vi "Pasive Response to IP & Port.vi"(8 "error in (no error)":errorcluster, 10 "Response":string, 11 "FTP in":refnum<class "FTP.lvclass">) -> (0 "error out":errorcluster, 1 "Port":u16, 2 "IP":u32 format="%x", 3 "FTP out":refnum<class "FTP.lvclass">)   [LabVIEW 2020, in "FTP.lvlib" / "FTP.lvclass"]
uses:
  FTP.lvclass
panel:
  out "array":u32[](array[numeric]) format="%x"
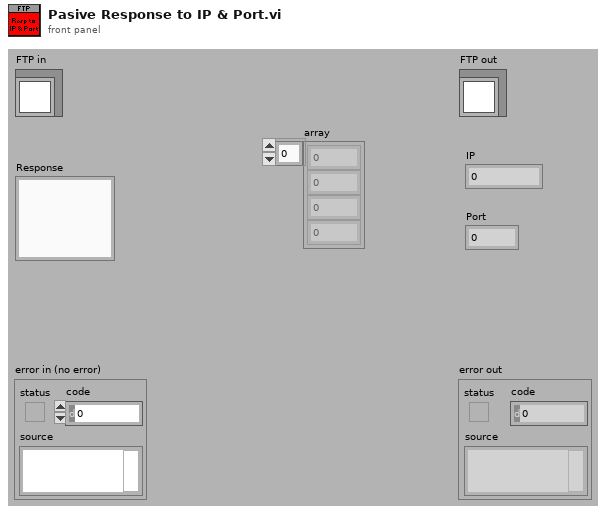
[diagram p1: front panel]
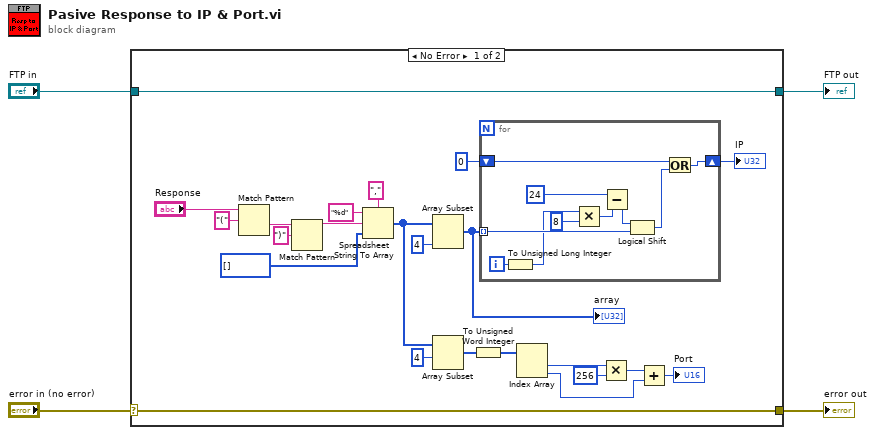
[diagram p0: block diagram]
diagram:
  n1 = case shown="No Error" "error in (no error)" {
    selector: "error in (no error)" -> [w26 w39]
    tunnel: [w26 w39] -> w3
    tunnel: [w27 w38] -> w1
    tunnel: "FTP in" -> [w27 w38]
    frame No Error {
      n2 = Match Pattern(string="Response", regular expression="(") -> (after substring=w25:string)  [unwired: 1 in, 3 out]
      n3 = Match Pattern(string=w25, regular expression=")") -> (before substring=w22:string)  [unwired: 1 in, 3 out]
      n4 = Spreadsheet String To Array(delimiter (Tab)=",", format string="%d", spreadsheet string=w22, array type (2D Dbl)=u32[] []) -> (array=w16:u32[])
      n5 = Array Subset(array=w16, length=4) -> (w7:u32[])  [unwired: 1 in]
      "array" <- w7
      n6 = Array Subset(array=w16, index=4) -> (w14:u32[])  [unwired: 1 in]
      n7 = To Unsigned Word Integer(number=w14) -> (unsigned 16bit integer=w5:u16[])
      n8 = for {
        tunnel: w7 -> [w37] mode=indexing
        shift-right: [w29] -> w6
        shift-left: u32 0 -> [w31]
        i -> [w34]
        n9 = To Unsigned Long Integer(number=w34) -> (unsigned 32bit integer=w28:u32)
        n10 = Multiply(x=w28, y=u32 8) -> (x*y=w35:u32)
        n11 = Subtract(x=u32 24 ("y"), y=w35) -> (x-y=w32:u32)
        n12 = Logical Shift(y=w32, x=w37) -> (x << y=w30:u32)
        n13 = Or(x=w31, y=w30) -> (x .or. y?=w29:u32)
      }
      "IP" <- w6
      n14 = Index Array(array=w5) -> (element #1=w13:u16, element #2=w10:u16)  [unwired: 2 in]
      n15 = Multiply(x=w13, y=u16 256) -> (x*y=w11:u16)
      n16 = Add(x=w11, y=w10) -> (x+y=→"Port":u16)
    }
    frame Error {
    }
  }
  "error out" <- w3
  "FTP out" <- w1
